vi "Automatic Mode.vi"(7 "Testing":bool, 11 "User Interface Cluster":T1={"Serial Settings"={"baud rate"=9600, "data bits"=8, "parity"=enum."None", "stop bits"=10, "flow control"=0}, "Serial Port"="", "Winding Distance (degrees)"=0.0, "Winding Speed"=0.0, "Dwell time (s)"=0.0, "Unwinding Distance (degrees)"=0.0, "Unwinding Speed"=0.0, "Output Data Path"=path "", "Sample Prefix:"="Applicator Test", "Sample Number:"=0, "Output Data Base Path"=path "C:/Users/Public/Data", "Auto-Increment Sample Number"=FALSE} {"Serial Settings"."flow control" items=["None"=0, "XON/XOFF"=1, "RTS/CTS"=2, "DTR/DSR"=4]; "Serial Settings"."stop bits" items=["1.0"=10, "1.5"=15, "2.0"=20]; "Serial Settings"."data bits" min=5 max=8 step=1; "Serial Settings"."baud rate" items=["75"=75, "110"=110, "134"=134, "150"=150, "300"=300, "600"=600, "1200"=1200, "1800"=1800, "2400"=2400, "4800"=4800, "7200"=7200, "9600"=9600, "14400"=14400, "19200"=19200, "28800"=28800, "38400"=38400, "56000"=56000, "57600"=57600, "115200"=115200, "128000"=128000, "230400"=230400]}) -> (2 "Output Data":dbl[][](array[numeric]), 3 "Test Complete":bool)   [LabVIEW 2019]
uses:
  Controls/User Interface Cluster.ctl
  Serial Comms/Serial - Settings.ctl
  Controls/Spring Test States.ctl
  Serial Comms/Serial Connection States.ctl
  <vilib>/Utility/error.llb/DialogType.ctl
  <vilib>/Utility/file.llb/Write Delimited Spreadsheet (string).vi
  <vilib>/Utility/file.llb/Write Delimited Spreadsheet (DBL).vi
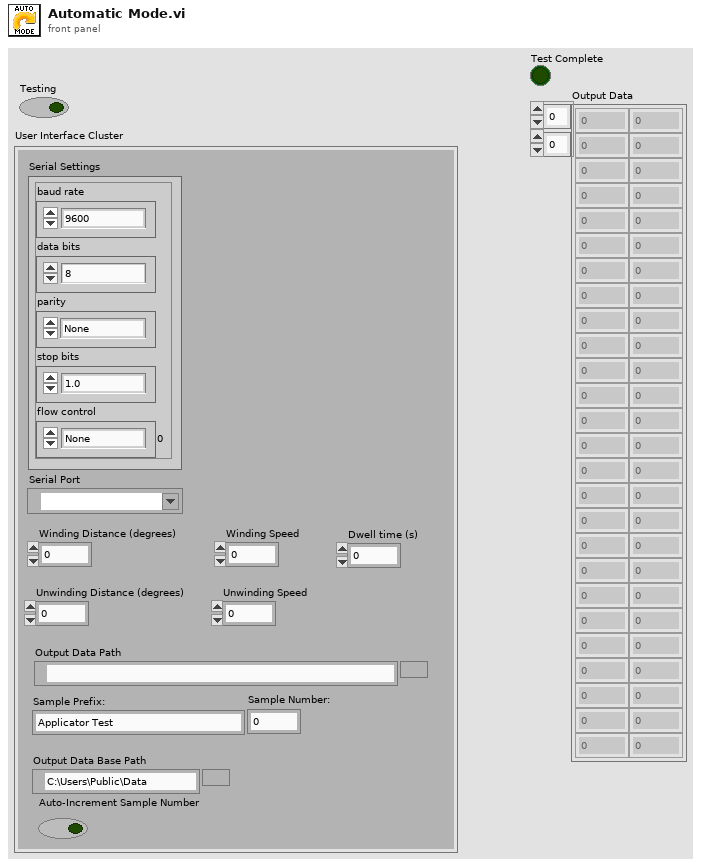
[diagram p1: front panel]
types:
  T1 = typedef "User Interface Cluster.ctl" = cluster{"Serial Settings":T2, "Serial Port":refnum<visa-resource-name>, "Winding Distance (degrees)":dbl, "Winding Speed":dbl, "Dwell time (s)":dbl, "Unwinding Distance (degrees)":dbl, "Unwinding Speed":dbl, "Output Data Path":path, "Sample Prefix:":string, "Sample Number:":u32, "Output Data Base Path":path, "Auto-Increment Sample Number":bool}
  T2 = typedef "Serial - Settings.ctl" = cluster{"baud rate":u32, "data bits":u16, "parity":enum16{"None", "Odd", "Even", "Mark", "Space"}, "stop bits":u16, "flow control":u16}
  T3 = typedef "Spring Test States.ctl" = enum16{"Idle", "Winding", "Start Winding Log", "Dwell & Log", "Unwind", "Start Unwinding Log", "Wait for Unwind", "Write to File", "Test Complete", "Stop"}
  T4 = typedef "Serial Connection States.ctl" = enum16{"Connect", "Get Connection", "Disconnect"}
  T5 = typedef "DialogType.ctl" = u16
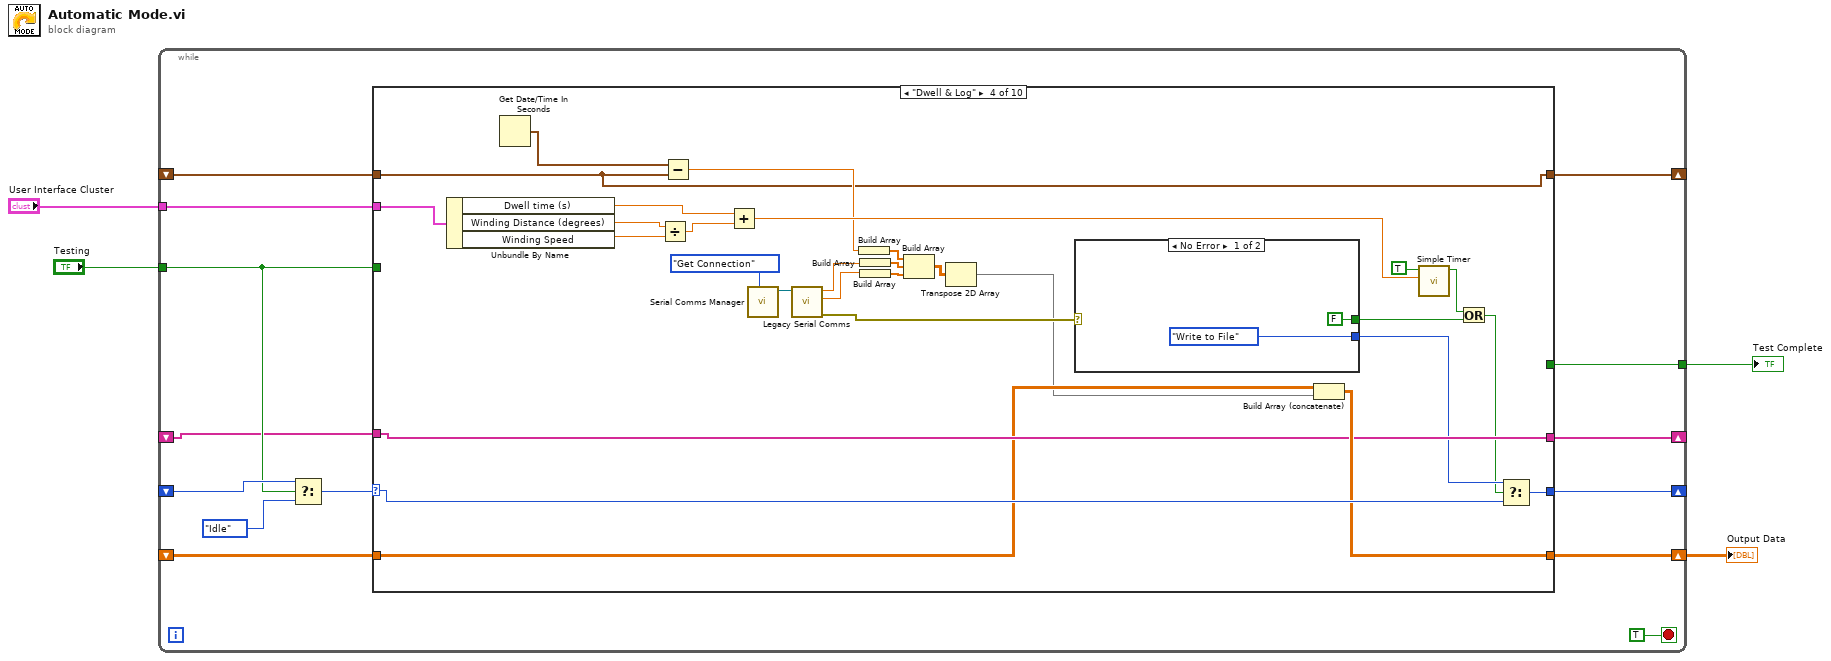
[diagram p0: block diagram]
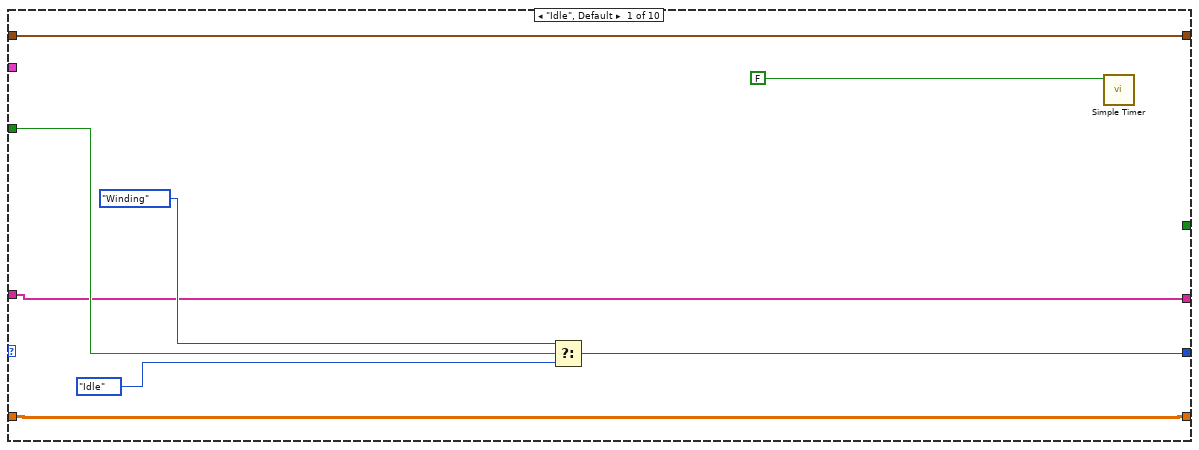
[diagram p2: hidden frame]
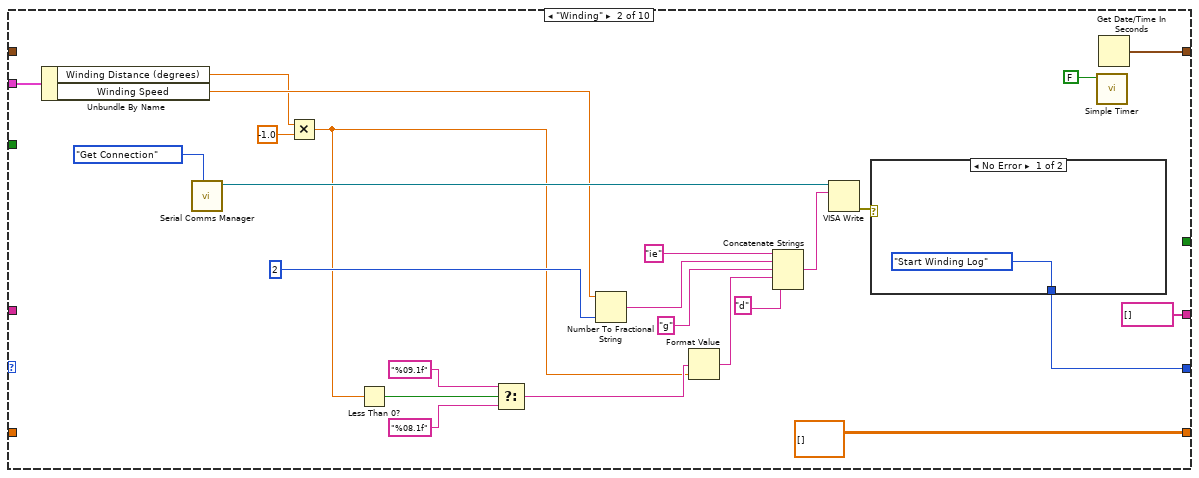
[diagram p3: hidden frame]
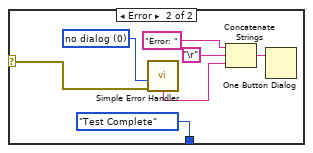
[diagram p4: hidden frame]
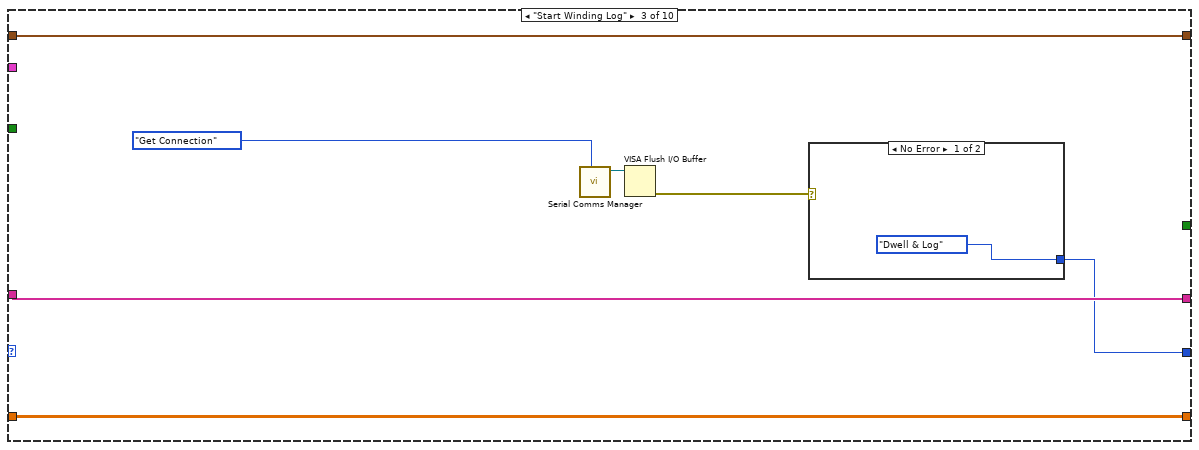
[diagram p5: hidden frame]
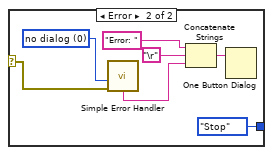
[diagram p6: hidden frame]
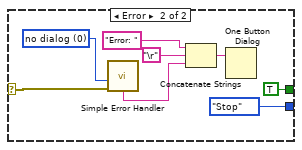
[diagram p7: hidden frame]
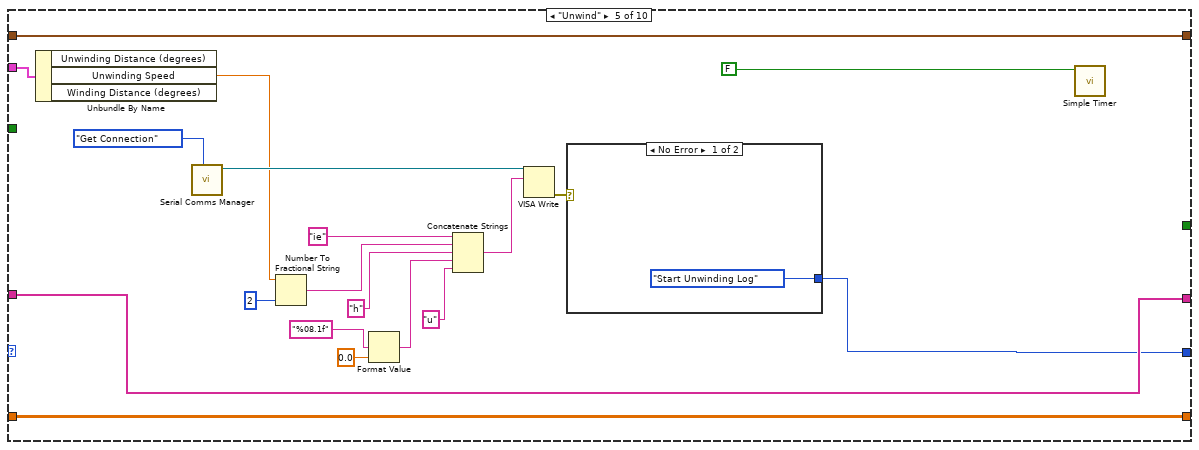
[diagram p8: hidden frame]
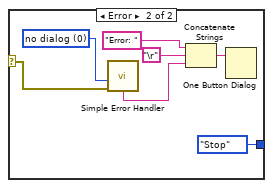
[diagram p9: hidden frame]
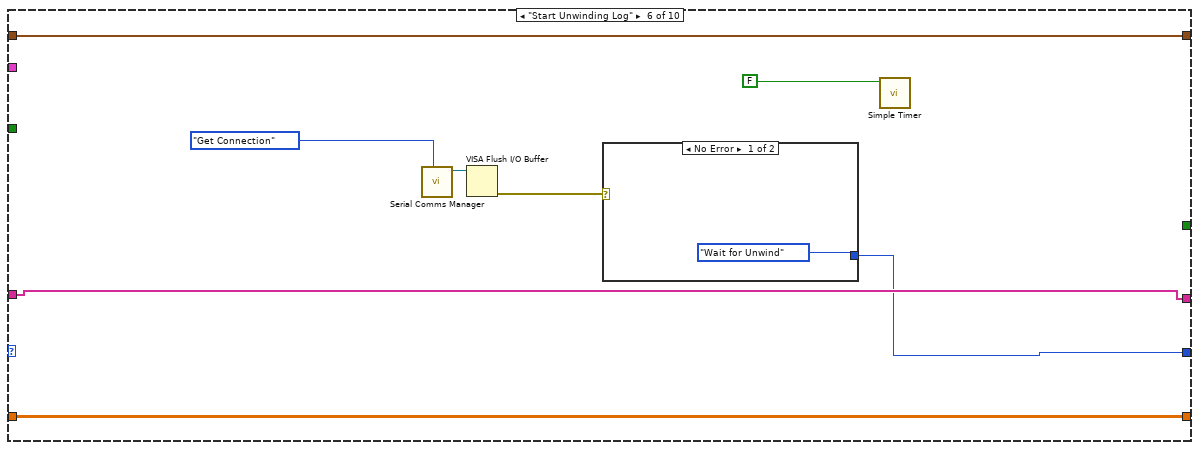
[diagram p10: hidden frame]
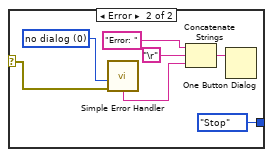
[diagram p11: hidden frame]
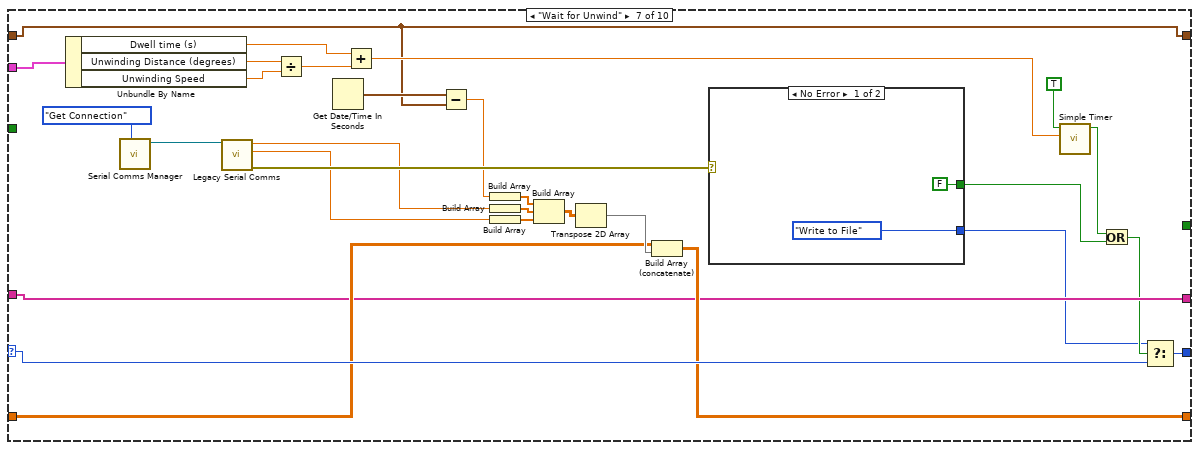
[diagram p12: hidden frame]
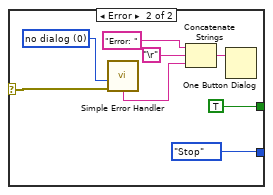
[diagram p13: hidden frame]
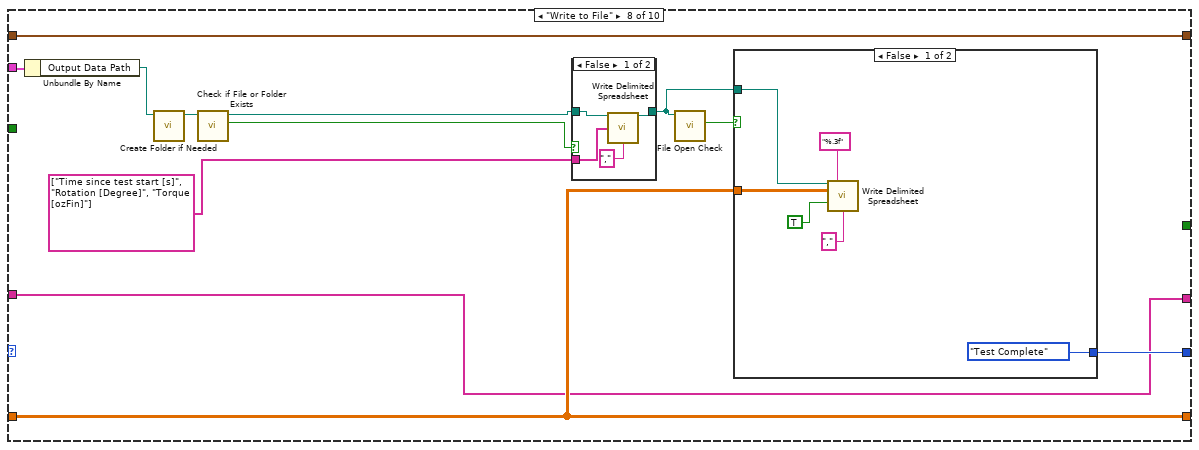
[diagram p14: hidden frame]
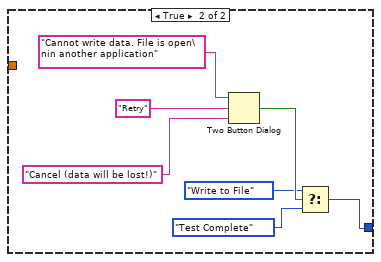
[diagram p16: hidden frame]
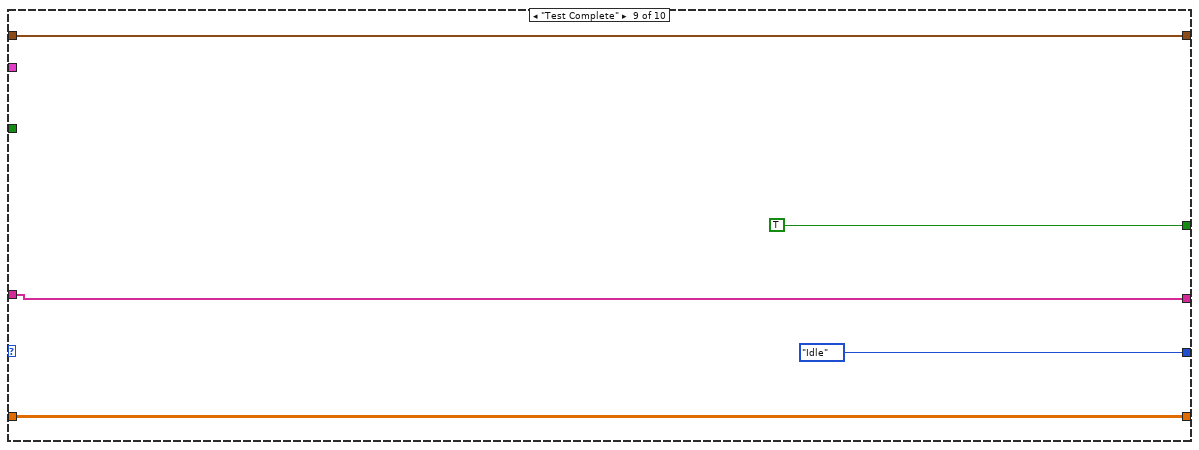
[diagram p17: hidden frame]
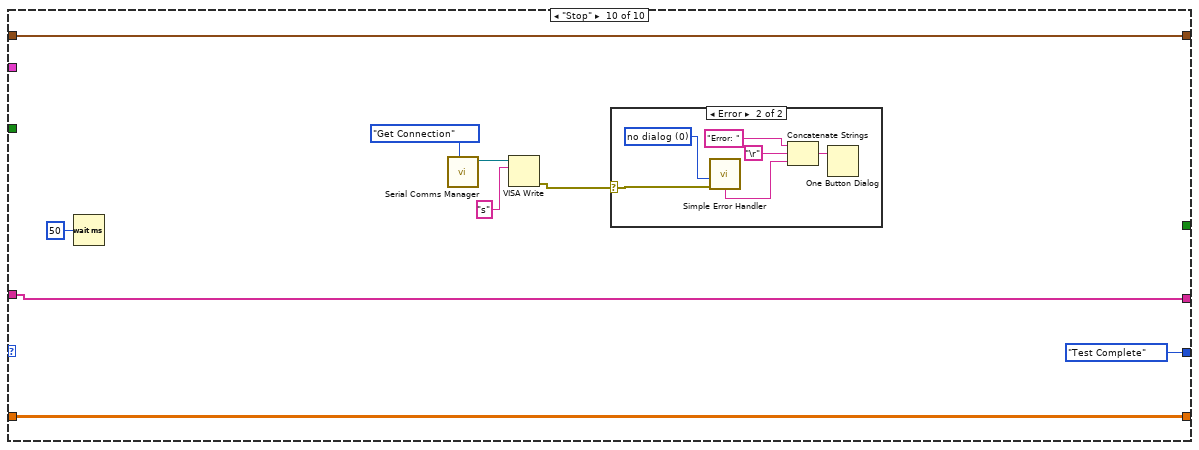
[diagram p18: hidden frame]
diagram:
  n1 = while {
    tunnel: "Testing" -> [w14]
    shift-right: [w13] -> _
    shift-left: _ -> [w17]
    tunnel: "User Interface Cluster" -> [w12]
    shift-right: [w10] -> w1
    shift-left: _ -> [w11]
    tunnel: [w9] -> w2
    shift-right: [w8] -> _
    shift-left: _ -> [w7]
    shift-right: [w6] -> _
    shift-left: _ -> [w5]
    stop <- TRUE stop-if-true
    n2 = Select(t=w17, s=w14, f=Spring_Test_States."Idle") -> (s? t:f=w15:T3)
    n3 = case shown="\"Dwell & Log\"" w15 {
      selector: w15 -> [_ _ _ w101 _ _ w183 _ _ _]
      tunnel: w14 -> [w26 _ _ _ _ _ _ _ _ _]
      tunnel: [w23 w28 w60 w100 w114 w141 w182 w203 Spring_Test_States."Idle" ("f") Spring_Test_States."Test Complete" ("t")] -> w13
      tunnel: w12 -> [_ w47 _ w99 w128 _ w181 w206 _ _]
      tunnel: w11 -> [w22 _ w63 w88 w117 w145 w175 w205 w229 w232]
      tunnel: [w22 dbl[][] [] w63 w97 w117 w145 w174 w205 w229 w232] -> w10
      tunnel: [_ _ _ _ _ _ _ _ TRUE _] -> w9
      tunnel: [w20 string[] [] w61 w90 w115 w142 w173 w196 w226 w234] -> w8
      tunnel: w7 -> [w20 _ w61 w90 w115 w142 w173 w196 w226 w234]
      tunnel: [w19 w27 w59 w74 w113 w140 w157 w195 w225 w230] -> w6
      tunnel: w5 -> [w19 _ w59 w74 w113 w140 w157 w195 w225 w230]
      frame "Idle", Default {
        n4 = Select(t=Spring_Test_States."Winding" ("f"), s=w26, f=Spring_Test_States."Idle") -> (s? t:f=w23:T3)
        n5 = call "Simple Timer.vi"("Timing?"=FALSE) -> ()  [unwired: 9 in, 2 out]
      }
      frame "Winding" {
        n6 = Unbundle By Name(w47) -> ("Winding Distance (degrees)"=w35:dbl, "Winding Speed"=w43:dbl)
        n7 = call "Serial Comms Manager.vi"("Action"=Serial_Connection_States."Get Connection") -> ("VISA resource name out"=w49:refnum<visa-resource-name>)  [unwired: 9 in, 1 out]
        n8 = Multiply(x=w35, y=-1.0) -> (x*y=w30:dbl)
        n9 = Less Than 0?(x=w30) -> (x < 0?=w29:bool)
        n10 = Select(t="%09.1f" ("format string"), s=w29, f="%08.1f" ("format string")) -> (s? t:f=w31:string)
        n11 = Number To Fractional String(number=w43, precision (6)=i16 2) -> (F-format string=w42:string)  [unwired: 2 in]
        n12 = Format Value(format string=w31, value (0)=w30) -> (output string=w40:string)  [unwired: 1 in]
        n13 = Concatenate Strings("ie", w42, "g" ("string"), w40, "d" ("string")) -> (w38:string)
        n14 = VISA Write(VISA resource name=w49, write buffer=w38) -> (error out=w48:errorcluster)  [unwired: 1 in, 2 out]
        n15 = case shown="No Error" w48 {
          selector: w48 -> [_ w57]
          tunnel: [Spring_Test_States."Start Winding Log" ("f") Spring_Test_States."Test Complete" ("f")] -> w28
          frame No Error {
          }
          frame Error {
            w58 = T5 0 items=["no dialog", "OK message", "continue or stop message", "OK message + warnings", "continue/stop + warnings"] ("type of dialog (OK msg:1)")
            n16 = call <vilib>:"Simple Error Handler.vi"("type of dialog (OK msg:1)"=w58, "error in (no error)"=w57) -> ("message"=w53:string)  [unwired: 3 in, 4 out]
            n17 = Concatenate Strings("Error: ", "\r", w53) -> (w54:string)
            n18 = One Button Dialog(message=w54) -> ()  [unwired: 1 in, 1 out]
          }
        }
        n19 = call "Simple Timer.vi"("Timing?"=FALSE) -> ()  [unwired: 9 in, 2 out]
        n20 = Get Date/Time In Seconds() -> (seconds since 1Jan1904=w27:timestamp)
      }
      frame "Start Winding Log" {
        n21 = call "Serial Comms Manager.vi"("Action"=Serial_Connection_States."Get Connection") -> ("VISA resource name out"=w64:refnum<visa-resource-name>)  [unwired: 9 in, 1 out]
        n22 = VISA Flush I/O Buffer(VISA resource name=w64) -> (error out=w62:errorcluster)  [unwired: 2 in, 1 out]
        n23 = case shown="No Error" w62 {
          selector: w62 -> [_ w72]
          tunnel: [Spring_Test_States."Dwell & Log" ("f") Spring_Test_States."Stop" ("f")] -> w60
          frame No Error {
          }
          frame Error {
            w73 = T5 0 items=["no dialog", "OK message", "continue or stop message", "OK message + warnings", "continue/stop + warnings"] ("type of dialog (OK msg:1)")
            n24 = call <vilib>:"Simple Error Handler.vi"("type of dialog (OK msg:1)"=w73, "error in (no error)"=w72) -> ("message"=w68:string)  [unwired: 3 in, 4 out]
            n25 = Concatenate Strings("Error: ", "\r", w68) -> (w69:string)
            n26 = One Button Dialog(message=w69) -> ()  [unwired: 1 in, 1 out]
          }
        }
      }
      frame "Dwell & Log" {
        n27 = Unbundle By Name(w99) -> ("Dwell time (s)"=w80:dbl, "Winding Distance (degrees)"=w82:dbl, "Winding Speed"=w81:dbl)
        n28 = Get Date/Time In Seconds() -> (seconds since 1Jan1904=w77:timestamp)
        n29 = Divide(x=w82, y=w81) -> (x/y=w79:dbl)
        n30 = Subtract(x=w77, y=w74) -> (x-y=w76:dbl)
        n31 = Add(x=w80, y=w79) -> (x+y=w78:dbl)
        n32 = call "Serial Comms Manager.vi"("Action"=Serial_Connection_States."Get Connection") -> ("VISA resource name out"=w96:refnum<visa-resource-name>)  [unwired: 9 in, 1 out]
        n33 = call "Legacy Serial Comms.vi"("VISA Refnum in"=w96) -> ("error out"=w89:errorcluster, "Numeric"=w91:dbl, "Numeric 2"=w92:dbl)  [unwired: 8 in]
        n34 = Build Array(w76) -> (w75:dbl[])
        n35 = Build Array(w92) -> (w95:dbl[])
        n36 = Build Array(w91) -> (w94:dbl[])
        n37 = Build Array(w75, w95, w94) -> (w93:dbl[][])
        n38 = Transpose 2D Array(2D array=w93) -> (transposed array=w87:dbl[][])
        n39 = case shown="No Error" w89 {
          selector: w89 -> [_ w111]
          tunnel: [Spring_Test_States."Write to File" ("t") Spring_Test_States."Stop" ("t")] -> w86
          tunnel: [FALSE ("Timing?") TRUE ("Timing?")] -> w83
          frame No Error {
          }
          frame Error {
            w112 = T5 0 items=["no dialog", "OK message", "continue or stop message", "OK message + warnings", "continue/stop + warnings"] ("type of dialog (OK msg:1)")
            n40 = call <vilib>:"Simple Error Handler.vi"("type of dialog (OK msg:1)"=w112, "error in (no error)"=w111) -> ("message"=w107:string)  [unwired: 3 in, 4 out]
            n41 = Concatenate Strings("Error: ", "\r", w107) -> (w108:string)
            n42 = One Button Dialog(message=w108) -> ()  [unwired: 1 in, 1 out]
          }
        }
        n43 = Build Array (concatenate) ("Data Buffer")(w88, w87) -> (w97:dbl[][])
        n44 = call "Simple Timer.vi"("Target [s]"=w78, "Timing?"=TRUE) -> ("Target Reached"=w85:bool)  [unwired: 8 in, 1 out]
        n45 = Or(x=w85, y=w83) -> (x .or. y?=w84:bool)
        n46 = Select(t=w86, s=w84, f=w101) -> (s? t:f=w100:T3)
      }
      frame "Unwind" {
        n47 = Unbundle By Name(w128) -> ("Unwinding Speed"=w125:dbl)  [unwired: 2 out]
        n48 = call "Serial Comms Manager.vi"("Action"=Serial_Connection_States."Get Connection") -> ("VISA resource name out"=w130:refnum<visa-resource-name>)  [unwired: 9 in, 1 out]
        n49 = Number To Fractional String(number=w125, precision (6)=i16 2) -> (F-format string=w124:string)  [unwired: 2 in]
        n50 = Format Value(format string="%08.1f", value (0)=0.0) -> (output string=w121:string)  [unwired: 1 in]
        n51 = Concatenate Strings("ie", w124, "h" ("string"), w121, "u" ("string")) -> (w119:string)
        n52 = VISA Write(VISA resource name=w130, write buffer=w119) -> (error out=w129:errorcluster)  [unwired: 1 in, 2 out]
        n53 = case shown="No Error" w129 {
          selector: w129 -> [_ w138]
          tunnel: [Spring_Test_States."Start Unwinding Log" ("f") Spring_Test_States."Stop" ("f")] -> w114
          frame No Error {
          }
          frame Error {
            w139 = T5 0 items=["no dialog", "OK message", "continue or stop message", "OK message + warnings", "continue/stop + warnings"] ("type of dialog (OK msg:1)")
            n54 = call <vilib>:"Simple Error Handler.vi"("type of dialog (OK msg:1)"=w139, "error in (no error)"=w138) -> ("message"=w134:string)  [unwired: 3 in, 4 out]
            n55 = Concatenate Strings("Error: ", "\r", w134) -> (w135:string)
            n56 = One Button Dialog(message=w135) -> ()  [unwired: 1 in, 1 out]
          }
        }
        n57 = call "Simple Timer.vi"("Timing?"=FALSE) -> ()  [unwired: 9 in, 2 out]
      }
      frame "Start Unwinding Log" {
        n58 = call "Serial Comms Manager.vi"("Action"=Serial_Connection_States."Get Connection") -> ("VISA resource name out"=w146:refnum<visa-resource-name>)  [unwired: 9 in, 1 out]
        n59 = VISA Flush I/O Buffer(VISA resource name=w146) -> (error out=w143:errorcluster)  [unwired: 2 in, 1 out]
        n60 = case shown="No Error" w143 {
          selector: w143 -> [_ w154]
          tunnel: [Spring_Test_States."Wait for Unwind" ("f") Spring_Test_States."Stop" ("f")] -> w141
          frame No Error {
          }
          frame Error {
            w155 = T5 0 items=["no dialog", "OK message", "continue or stop message", "OK message + warnings", "continue/stop + warnings"] ("type of dialog (OK msg:1)")
            n61 = call <vilib>:"Simple Error Handler.vi"("type of dialog (OK msg:1)"=w155, "error in (no error)"=w154) -> ("message"=w150:string)  [unwired: 3 in, 4 out]
            n62 = Concatenate Strings("Error: ", "\r", w150) -> (w151:string)
            n63 = One Button Dialog(message=w151) -> ()  [unwired: 1 in, 1 out]
          }
        }
        n64 = call "Simple Timer.vi"("Timing?"=FALSE) -> ()  [unwired: 9 in, 2 out]
      }
      frame "Wait for Unwind" {
        n65 = Unbundle By Name(w181) -> ("Dwell time (s)"=w162:dbl, "Unwinding Distance (degrees)"=w164:dbl, "Unwinding Speed"=w163:dbl)
        n66 = call "Serial Comms Manager.vi"("Action"=Serial_Connection_States."Get Connection") -> ("VISA resource name out"=w172:refnum<visa-resource-name>)  [unwired: 9 in, 1 out]
        n67 = call "Legacy Serial Comms.vi"("VISA Refnum in"=w172) -> ("error out"=w171:errorcluster, "Numeric"=w169:dbl, "Numeric 2"=w170:dbl)  [unwired: 8 in]
        n68 = Divide(x=w164, y=w163) -> (x/y=w161:dbl)
        n69 = Get Date/Time In Seconds() -> (seconds since 1Jan1904=w158:timestamp)
        n70 = Add(x=w162, y=w161) -> (x+y=w160:dbl)
        n71 = Subtract(x=w158, y=w157) -> (x-y=w156:dbl)
        n72 = Build Array(w156) -> (w159:dbl[])
        n73 = Build Array(w170) -> (w178:dbl[])
        n74 = Build Array(w169) -> (w179:dbl[])
        n75 = Build Array(w159, w178, w179) -> (w180:dbl[][])
        n76 = Transpose 2D Array(2D array=w180) -> (transposed array=w176:dbl[][])
        n77 = Build Array (concatenate) ("Data Buffer")(w175, w176) -> (w174:dbl[][])
        n78 = case shown="No Error" w171 {
          selector: w171 -> [_ w193]
          tunnel: [FALSE ("Timing?") TRUE ("Timing?")] -> w166
          tunnel: [Spring_Test_States."Write to File" ("t") Spring_Test_States."Stop" ("t")] -> w165
          frame No Error {
          }
          frame Error {
            w194 = T5 0 items=["no dialog", "OK message", "continue or stop message", "OK message + warnings", "continue/stop + warnings"] ("type of dialog (OK msg:1)")
            n79 = call <vilib>:"Simple Error Handler.vi"("type of dialog (OK msg:1)"=w194, "error in (no error)"=w193) -> ("message"=w189:string)  [unwired: 3 in, 4 out]
            n80 = Concatenate Strings("Error: ", "\r", w189) -> (w190:string)
            n81 = One Button Dialog(message=w190) -> ()  [unwired: 1 in, 1 out]
          }
        }
        n82 = call "Simple Timer.vi"("Target [s]"=w160, "Timing?"=TRUE) -> ("Target Reached"=w168:bool)  [unwired: 8 in, 1 out]
        n83 = Or(x=w168, y=w166) -> (x .or. y?=w167:bool)
        n84 = Select(t=w165, s=w167, f=w183) -> (s? t:f=w182:T3)
      }
      frame "Write to File" {
        n85 = Unbundle By Name(w206) -> ("Output Data Path"=w204:path)
        n86 = call "Create Folder if Needed.vi"("Settings File Path"=w204) -> ("File Path Out"=w201:path)  [unwired: 10 in]
        n87 = call <vilib>:"Check if File or Folder Exists.vi"("path"=w201) -> ("file or folder exists?"=w200:bool, "dup path"=w199:path)  [unwired: 8 in, 1 out]
        n88 = case shown="False" w200 {
          tunnel: [w209 w211] -> w197
          tunnel: w199 -> [w210 w211]
          tunnel: string[] ["Time since test start [s]", "Rotation [Degree]", "Torque [ozFin]"] -> [w208 _]
          frame False {
            n89 = call-poly <vilib>:"Write Delimited Spreadsheet.vi"("file path (dialog if empty)"=w210, "1D data"=w208, "delimiter (\\t)"=",") -> ("new file path (Not A Path if cancelled)"=w209:path)  [unwired: 11 in, 1 out]
          }
          frame True {
          }
        }
        n90 = call "File Open Check.vi"("File Path"=w197) -> ("File is open in another application"=w202:bool)  [unwired: 9 in, 1 out]
        n91 = case shown="False" w202 {
          tunnel: w205 -> [w214 _]
          tunnel: [Spring_Test_States."Test Complete" ("f") w218] -> w203
          tunnel: w197 -> [w212 _]
          frame False {
            n92 = call-poly <vilib>:"Write Delimited Spreadsheet.vi"("file path (dialog if empty)"=w212, "format (%.3f)"="%.3f", "2D data"=w214, "append to file? (new file:F)"=TRUE, "delimiter (\\t)"=",") -> ()  [unwired: 9 in, 2 out]
          }
          frame True {
            n93 = Two Button Dialog(message="Cannot write data. File is open\nin another application", 1:"Cancel (data will be lost!)" ("F button name (\"Cancel\")"), 2:"Retry" ("T button name (\"OK\")")) -> (T button?=w221:bool)
            n94 = Select(t=Spring_Test_States."Write to File" ("f"), s=w221, f=Spring_Test_States."Test Complete") -> (s? t:f=w218:T3)
          }
        }
      }
      frame "Test Complete" {
      }
      frame "Stop" {
        n95 = Wait (ms)(milliseconds to wait=u32 50) -> ()  [unwired: 1 out]
        n96 = call "Serial Comms Manager.vi"("Action"=Serial_Connection_States."Get Connection") -> ("VISA resource name out"=w236:refnum<visa-resource-name>)  [unwired: 9 in, 1 out]
        n97 = VISA Write(VISA resource name=w236, write buffer="s") -> (error out=w233:errorcluster)  [unwired: 1 in, 2 out]
        n98 = case shown="Error" w233 {
          selector: w233 -> [_ w243]
          frame No Error {
          }
          frame Error {
            w244 = T5 0 items=["no dialog", "OK message", "continue or stop message", "OK message + warnings", "continue/stop + warnings"] ("type of dialog (OK msg:1)")
            n99 = call <vilib>:"Simple Error Handler.vi"("type of dialog (OK msg:1)"=w244, "error in (no error)"=w243) -> ("message"=w239:string)  [unwired: 3 in, 4 out]
            n100 = Concatenate Strings("Error: ", "\r", w239) -> (w240:string)
            n101 = One Button Dialog(message=w240) -> ()  [unwired: 1 in, 1 out]
          }
        }
      }
    }
  }
  "Test Complete" <- w2
  "Output Data" <- w1
